vi "Demo.vi"() -> ()   [LabVIEW 2021, in "UserEvent.lvlib"]
uses:
  UserEvent.lvlib
  a2408f8a-ddaa-4cbd-a54b-6b90a31d1fb1.vi
  2cda9ea2-0308-4cd9-9462-b881e2ed9209.vi
  59c65931-af44-41da-b623-b7e15c6788b5.vi
  21db829a-ce00-46c8-a8f8-4cce8163bba9.vi
  2868a04d-7363-4581-9b2c-7f370ceed1d7.vi
  SubVIs/Map.vi
panel:
  out "User Event Name":string
  out "ms Elapsed":u32
  out "Inc":i32
  out "Error":errorcluster
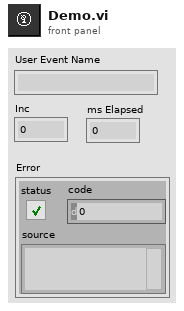
[diagram p1: front panel]
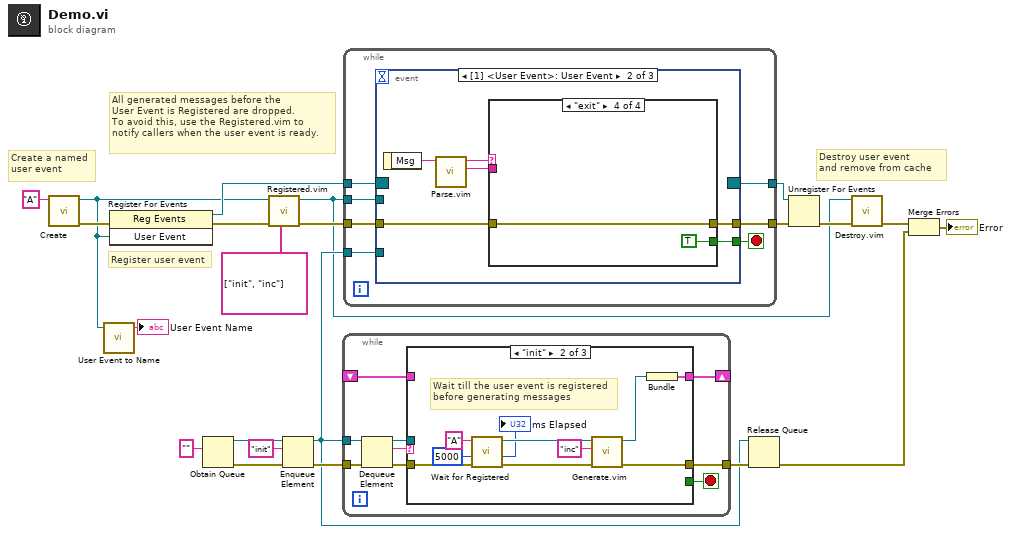
[diagram p0: block diagram]
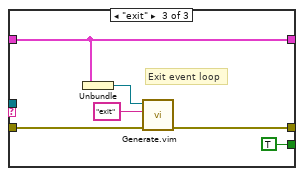
[diagram p3: hidden frame]
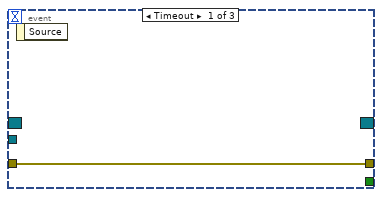
[diagram p4: hidden frame]
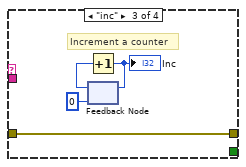
[diagram p7: hidden frame]
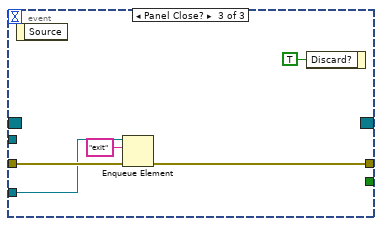
[diagram p8: hidden frame]
diagram:
  # "Destroy user event\nand remove from cache"
  # "Register user event"
  # "Create a named\nuser event"
  # "All generated messages before the\nUser Event is Registered are dropped.\nTo avoid this, use the Registered.vim to\nnotify callers when the user event is ready."
  n1 = call "Create.vi"("User Event Name (\"\"=Unnamed)"="A" ("User Event Name (\"\"=Unnamed)")) -> ("error out"=w22:errorcluster, "User Event"=w2:refnum<user-event>)  [unwired: 7 in, 2 out]
  n2 = call "User Event to Name.vi"("User Event"=w2) -> ("User Event Name"=→"User Event Name":string)  [unwired: 6 in, 2 out]
  n3 = register-events(error in=w22, w2) -> (reference out=w16:refnum<event-registration>, error out=w15:errorcluster)  [unwired: 1 in]
  n4 = Obtain Queue(element data type="") -> (queue out=w11:refnum<queue>, error out=w10:errorcluster)  [unwired: 4 in, 1 out]
  n5 = call "Registered.vim"("Messages"=string[] ["init", "inc"], "error in (no error)"=w15, "User Event in"=w2) -> ("error out"=w14:errorcluster, "User Event"=w3:refnum<user-event>)  [unwired: 7 in]
  n6 = Enqueue Element(queue=w11, element="init", error in (no error)=w10) -> (queue out=w4:refnum<queue>, error out=w8:errorcluster)  [unwired: 1 in, 1 out]
  n7 = while {
    tunnel: w4 -> [w31]
    tunnel: w8 -> [w30]
    tunnel: [w26] -> w7
    shift-right: [w24] -> _
    shift-left: _ -> [w23]
    stop <- w25 stop-if-true
    n8 = Dequeue Element(queue=w31, error in (no error)=w30) -> (queue out=w28:refnum<queue>, element=w29:string, error out=w27:errorcluster)  [unwired: 1 in, 1 out]
    n9 = case shown="\"init\"" w29 {
      tunnel: w28 -> [_ _ _]
      tunnel: w27 -> [w33 w43 w46]
      tunnel: [w33 w36 w47] -> w26
      tunnel: [_ _ TRUE] -> w25
      tunnel: [w32 w40 w45] -> w24
      tunnel: w23 -> [w32 _ w45]
      frame Default {
      }
      frame "init" {
        # "Wait till the user event is registered\nbefore generating messages"
        n10 = call "Wait for Registered.vi"("error in (no error)"=w43, "ms Timeout (5000)"=u32 5000, "User Event Name"="A") -> ("error out"=w37:errorcluster, "ms Elapsed"=→"ms Elapsed":u32, "User Event"=w39:refnum<user-event>)  [unwired: 6 in]
        n11 = call "Generate.vim"("error in (no error)"=w37, "Message"="inc", "User Event in"=w39) -> ("error out"=w36:errorcluster, "User Event"=w38:refnum<user-event>)  [unwired: 7 in]
        n12 = Bundle("User Event"=w38) -> (w40:cluster{"User Event":refnum<user-event>})  [unwired: 1 in]
      }
      frame "exit" {
        # "Exit event loop"
        n13 = Unbundle(w45) -> ("User Event"=w44:refnum<user-event>)
        n14 = call "Generate.vim"("error in (no error)"=w46, "Message"="exit", "User Event in"=w44) -> ("error out"=w47:errorcluster)  [unwired: 7 in, 1 out]
      }
    }
  }
  n15 = while {
    tunnel: [w56] -> w19
    tunnel: w14 -> [w55]
    tunnel: w16 -> [w54]
    tunnel: [w53] -> w20
    tunnel: w3 -> [w52]
    tunnel: w4 -> [w50]
    stop <- w51 stop-if-true
    n16 = event shown="[1] <User Event>: User Event" {
      selector: w54 -> [_ _ _]
      dyn-events: [_ _ _] -> w53
      timeout: _ -> [_ _ _]
      tunnel: [w57 w63 w74] -> w56
      tunnel: w55 -> [w57 w62 w75]
      tunnel: w52 -> [_ _ _]
      tunnel: [_ w58 _] -> w51
      tunnel: w50 -> [_ _ w73]
      event Timeout {
        n17 = event-data() -> ()  [unwired: 1 in, 1 out]
      }
      event User Event {
        n18 = event-data() -> ("Msg"=w61:string)  [unwired: 1 in]
        n19 = call "Parse.vim"("Msg"=w61) -> ("Data out"=w59:string, "Message out"=w60:string)  [unwired: 9 in]
        n20 = case shown="\"exit\"" w60 {
          tunnel: [w64 w65 w69 w71] -> w63
          tunnel: w62 -> [w64 w65 w69 w71]
          tunnel: w59 -> [_ _ _ _]
          tunnel: [_ _ _ TRUE] -> w58
          frame Default {
          }
          frame "init" {
          }
          frame "inc" {
            # "Increment a counter"
            n21 = feedback #1(0) -> (w67:i32)
            n22 = Increment(x=w67) -> (x+1=w66:i32)
            "Inc" <- w66
            n23 = feedback-in #1(w66) -> ()
          }
          frame "exit" {
          }
        }
      }
      event Panel Close? {
        n24 = event-data() -> ()  [unwired: 1 in, 1 out]
        n25 = Enqueue Element(queue=w73, element="exit", error in (no error)=w75) -> (error out=w74:errorcluster)  [unwired: 1 in, 2 out]
        n26 = event-data("Discard?"=TRUE) -> ()  [unwired: 1 in, 1 out]
      }
    }
  }
  n27 = Release Queue(queue=w4, error in (no error)=w7) -> (error out=w5:errorcluster)  [unwired: 1 in, 2 out]
  n28 = Unregister For Events(event registration refnum=w20, error in=w19) -> (error out=w18:errorcluster)
  n29 = call "Destroy.vim"("error in (no error)"=w18, "User Event in"=w3) -> ("error out"=w17:errorcluster)  [unwired: 8 in, 1 out]
  n30 = Merge Errors(w17, w5) -> (→"Error":errorcluster)
